vi "Subvi pixel clock gate.vi"(5 "Nmax lines":u16, 7 "Start_acquisition":bool, 11 "Pixel clock/line clock change":T1) -> (0 "Line gate":bool, 3 "Gated pixel clock change":bool, 4 "Pretrigger":bool)   [LabVIEW 2017]
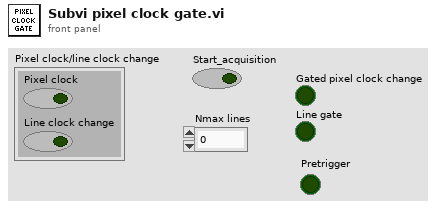
[diagram p1: front panel]
types:
  T1 = cluster{"Pixel clock":bool, "Line clock change":bool}
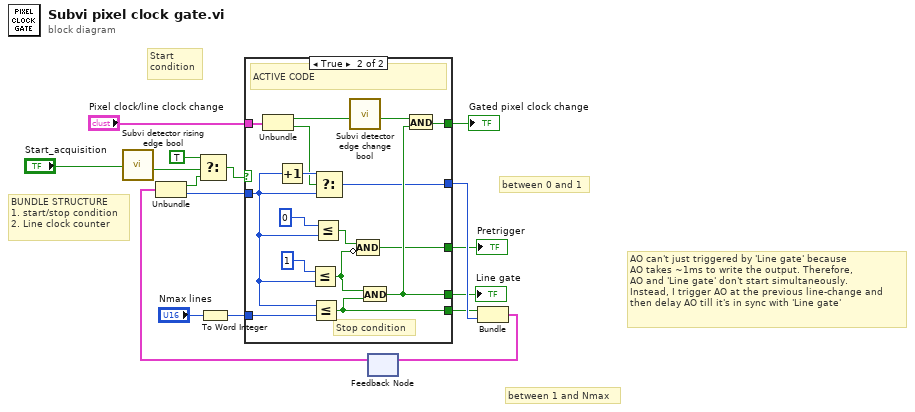
[diagram p0: block diagram]
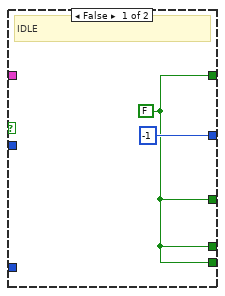
[diagram p2: hidden frame]
diagram:
  # "between 1 and Nmax"
  # "AO can't just triggered by 'Line gate' because\nAO takes ~1ms to write the output. Therefore,\nAO and 'Line gate' don't start simultaneously.\nInstead, I trigger AO at the previous line-change and\nthen delay AO till it's in sync with 'Line gate'"
  # "between 0 and 1"
  # "Start\ncondition"
  # "BUNDLE STRUCTURE\n1. start/stop condition\n2. Line clock counter"
  n1 = call "Subvi detector rising edge bool.vi"("Input"="Start_acquisition") -> ("Output"=w6:bool)  [unwired: 10 in]
  n2 = To Word Integer(number="Nmax lines") -> (16bit integer=w1:i16)
  n3 = feedback #1() -> (w14:cluster{bool, i16})  [unwired: 1 in]
  n4 = Unbundle(w14) -> (w15:bool, w16:i16)
  n5 = Select(t=TRUE, s=w6, f=w15) -> (s? t:f=w10:bool)
  n6 = case shown="True" w10 {
    tunnel: [w17 w28] -> w11
    tunnel: w16 -> [_ w23]
    tunnel: [i16 -1 w24] -> w12
    tunnel: "Pixel clock/line clock change" -> [_ w34]
    tunnel: [w17 w33] -> w5
    tunnel: [w17 w25] -> w4
    tunnel: w1 -> [_ w26]
    tunnel: [w17 w19] -> w2
    frame False {
      w17 = FALSE
      # "IDLE"
    }
    frame True {
      # "Stop condition"
      # "ACTIVE CODE"
      n7 = Unbundle(w34) -> ("Pixel clock"=w29:bool, "Line clock change"=w27:bool)
      n8 = Increment(x=w23) -> (x+1=w32:i16)
      n9 = Less Or Equal?(x=i16 1 ("Min"), y=w23) -> (x <= y?=w20:bool)
      n10 = Less Or Equal?(x=w23, y=w26) -> (x <= y?=w28:bool)
      n11 = Less Or Equal?(x=i16 0, y=w23) -> (x <= y?=w21:bool)
      n12 = Select(t=w32, s=w27, f=w23) -> (s? t:f=w24:i16)
      n13 = call "Subvi detector edge change bool.vi"("Input"=w29) -> ("Output"=w30:bool)  [unwired: 8 in]
      n14 = Compound Arithmetic op=AND(w21, invert w20) -> (w19:bool)
      n15 = And(x=w20, y=w28) -> (x .and. y?=w25:bool)
      n16 = And(x=w30, y=w25) -> (x .and. y?=w33:bool)
    }
  }
  "Gated pixel clock change" <- w5
  "Line gate" <- w4
  "Pretrigger" <- w2
  n17 = Bundle(w11, w12) -> (w13:cluster{bool, i16})  [unwired: 1 in]
  n18 = feedback-in #1(w13) -> ()
